vi "Reader_Regular DatTypes.vi"() -> ()   [LabVIEW 2018]
uses:
  NiFpga.dll
panel:
  out "Value":dbl
  out "error out":errorcluster
  in  "Error In":errorcluster
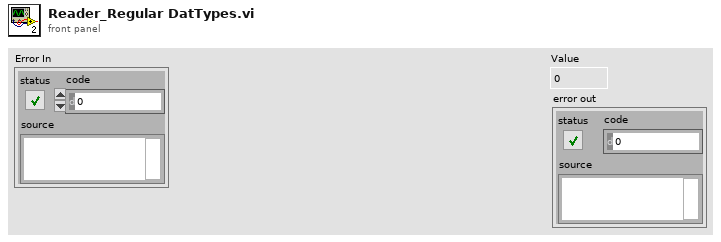
[diagram p1: front panel]
types:
  T1 = cluster{"Delta":dbl, "Word Length":u32, "Signed":bool, "offset":i32, "Name":string, "base address":i32}[]
  T2 = cluster{"Delta":dbl, "Word Length":u32, "Signed":bool, "offset":i32, "Name":string, "base address":i32}
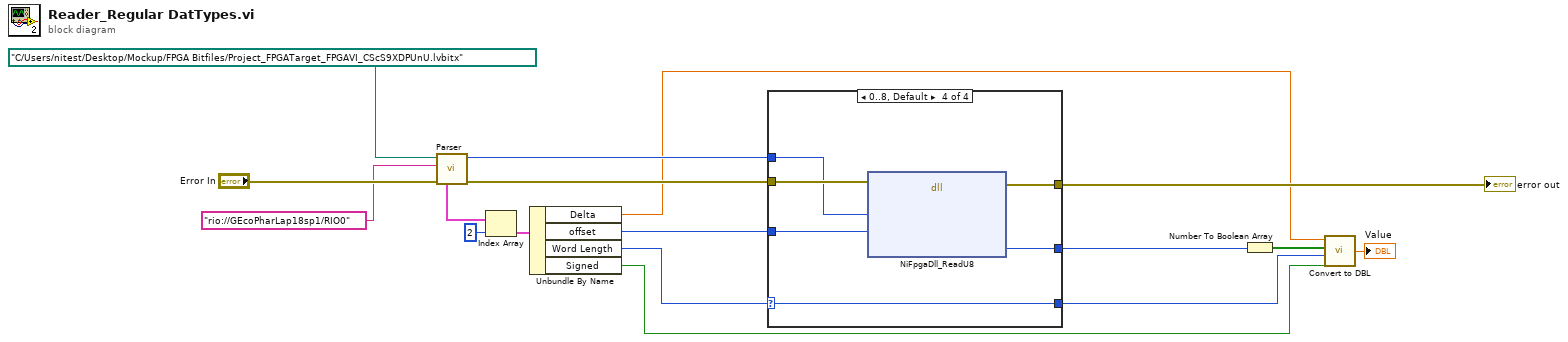
[diagram p0: block diagram]
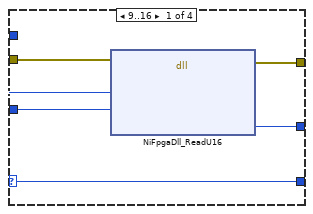
[diagram p2: hidden frame]
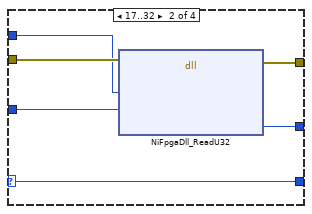
[diagram p3: hidden frame]
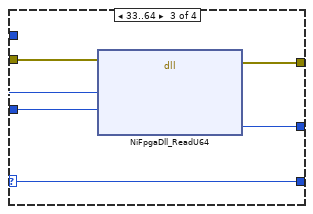
[diagram p4: hidden frame]
diagram:
  n1 = call "Parser.vi"("error in (no error)"="Error In", "RIO device address"="rio://GEcoPharLap18sp1/RIO0" ("Device address"), "bitfile path"=path "C:/Users/nitest/Desktop/Mockup/FPGA Bitfiles/Project_FPGATarget_FPGAVI_CScS9XDPUnU.lvbitx" ("Bitfile path")) -> ("error out"=w10:errorcluster, "FXP channels out"=w7:T1, "session out"=w8:u64)  [unwired: 6 in]
  n2 = Index Array(array=w7, index=2) -> (element=w5:T2)
  n3 = Unbundle By Name(w5) -> ("Delta"=w1:dbl, "offset"=w4:i32, "Word Length"=w3:u32, "Signed"=w2:bool)
  n4 = case shown="0..8, Default" w3 {
    selector: w3 -> [w21 w27 w33 w39]
    tunnel: [w23 w28 w35 w41] -> w17
    tunnel: [w22 w29 w34 w40] -> w16
    tunnel: [w21 w27 w33 w39] -> w13
    tunnel: w10 -> [w20 w26 w32 w38]
    tunnel: w8 -> [w18 w24 w31 w37]
    tunnel: w4 -> [w19 w25 w30 w36]
    frame 9..16 {
      n5 = dll-call lib="NiFpga.*" fn="NiFpgaDll_ReadU16"(error in=w20, "session"=w18, "offset"=w19) -> (error out=w23:errorcluster, "value"=w22:u8)  [unwired: 6 in, 1 out]
    }
    frame 17..32 {
      n6 = dll-call lib="NiFpga.*" fn="NiFpgaDll_ReadU32"(error in=w26, "session"=w24, "offset"=w25) -> (error out=w28:errorcluster, "value"=w29:u8)  [unwired: 6 in, 1 out]
    }
    frame 33..64 {
      n7 = dll-call lib="NiFpga.*" fn="NiFpgaDll_ReadU64"(error in=w32, "session"=w31, "offset"=w30) -> (error out=w35:errorcluster, "value"=w34:u8)  [unwired: 6 in, 1 out]
    }
    frame 0..8, Default {
      n8 = dll-call lib="NiFpga.*" fn="NiFpgaDll_ReadU8"(error in=w38, "session"=w37, "offset"=w36) -> (error out=w41:errorcluster, "value"=w40:u8)  [unwired: 6 in, 1 out]
    }
  }
  "error out" <- w17
  n9 = Number To Boolean Array(number=w16) -> (Boolean array=w15:bool[])
  n10 = call "Convert to DBL.vi"("Signed?"=w2, "Word Length"=w13, "Data"=w15, "Delta"=w1) -> ("x*y"=→"Value":dbl)
